vi "Find Abberation Excel Files_SLM.vi"() -> (0 "Ring Menu":cluster{"result string":string, i32}[](array[cluster]), 3 "Abberation File Paths":path[](array[path]))   [LabVIEW 2014]
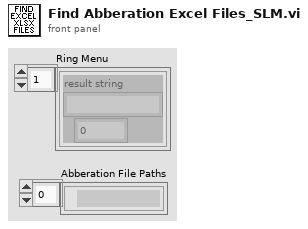
[diagram p1: front panel]
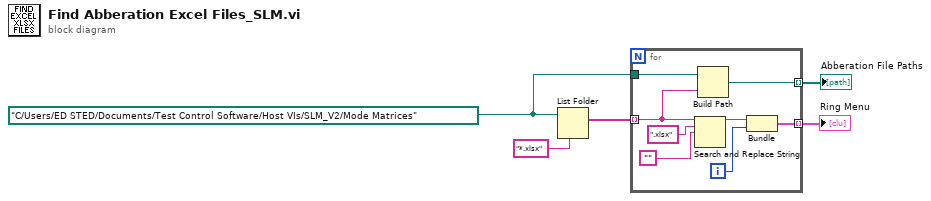
[diagram p0: block diagram]
diagram:
  w1 = path "C:/Users/ED STED/Documents/Test Control Software/Host VIs/SLM_V2/Mode Matrices" ("path")
  n1 = List Folder(path=w1, pattern="*.xlsx") -> (filenames=w5:string[])  [unwired: 2 in, 3 out]
  n2 = for {
    tunnel: w5 -> [w7] mode=indexing
    tunnel: [w9] -> w4 mode=indexing
    tunnel: w1 -> [w8]
    tunnel: [w6] -> w3 mode=indexing
    i -> [w10]
    n3 = Search and Replace String(input string=w7, search string=".xlsx", replace string="") -> (result string=w11:string)  [unwired: 5 in, 3 out]
    n4 = Build Path(base path=w8, name or relative path=w7) -> (appended path=w6:path)
    n5 = Bundle("result string"=w11, w10) -> (w9:cluster{"result string":string, i32})  [unwired: 1 in]
  }
  "Ring Menu" <- w4
  "Abberation File Paths" <- w3
